vi "Autonomous Independent (1).vi"() -> ()   [LabVIEW 2017]
doc: "This VI is called when autonomous begins, and will automatically be terminated when autonomous ends. You can carry out timed or sensor driven robot movement independently without needing to return to the caller."
uses:
  <vilib>/Rock Robotics/WPI/ThirdParty/Sensors/navX/_TypeDefs/FRIC_navX_DeviceNumbersTypeDef.ctl
  Public/Documents/Cross The Road Electronics/Phoenix-LabVIEW/Motor Controller/Controls/CTRE_Phoenix_MotorControl_ControlMode.ctl
  <vilib>/Rock Robotics/WPI/Utilities/WPI_GetSetVariantRefNum.vi
  <vilib>/Rock Robotics/Network Tables/NT Read String.vi
  <vilib>/Rock Robotics/Network Tables/NT Write Numeric Array.vi
panel:
  out "error out":errorcluster
  out "Array":dbl[](array[numeric])
  out "Direction":string[](array[string])
  in  "Target Angle":dbl format="%#_13g"
  in  "Target Distance":dbl=500.0 format="%#_13g"
  # "Be sure to right-click and choose Data Operations>>Make Current Value default if you want to save the array values with the VI"
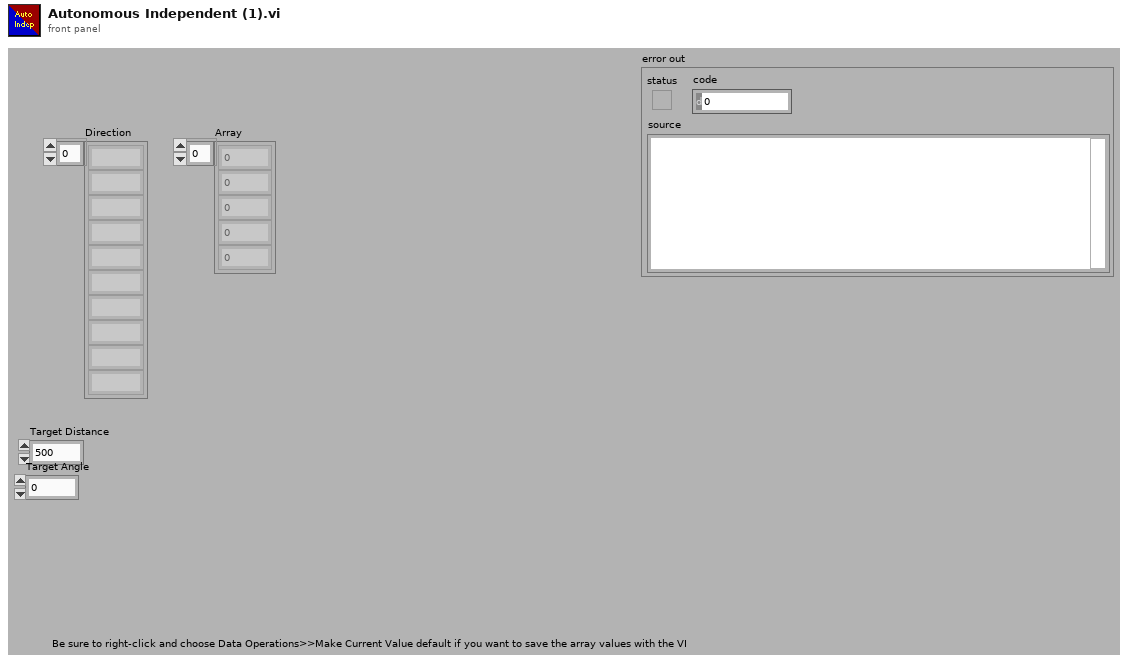
[diagram p1: front panel]
types:
  T1 = typedef "FRIC_navX_DeviceNumbersTypeDef.ctl" = enum16{"Dev0", "Dev1", "Dev2", "Dev3"}
  T2 = cluster{"Left Encoder":string, "Right Encoder":string, "Gyro Refnum":string, "Device Number":T1, "Right Refnum":string, "Left Refnum":string, "Right Intake":string, "Left Intake":string}
  T3 = typedef "WPI_JoystickDevRef.ctl" = cluster{"Device":T4}
  T4 = typedef "WPI_JoystickDeviceEnum.ctl" = enum16{"USB 0", "USB 1", "USB 2", "USB 3", "USB 4", "USB 5"}
  T5 = cluster{"Left Encoder":string, "Right Encoder":string, "Gyro Refnum":string, "Device Number":T1, "Right Refnum":string, "Left Refnum":string}
  T6 = cluster{"Left Encoder":string, "Right Encoder":string, "Gyro Refnum":string, "Device Number":T1, "Right Refnum":string, "Left Refnum":string, "Left Intake":string, "Right Intake":string}
  T7 = typedef "CTRE_Phoenix_MotorControl_ControlMode.ctl" = u16
  T8 = typedef "WPI_MotorControlDeviceRef.ctl" = cluster{"DeviceStatus":errorcluster, "Type":T9, "PWM":cluster{"PWM Channel":T10, "DeadBand":T11}, "CAN":cluster{"Device Number":u8, "SetOutput VI Ref":variant, "GetOutput VI Ref":variant, "Enable VI Ref":variant, "Disable VI Ref":variant, "Data":variant}, "Invert":bool, "DIO PWM":cluster{"PWM \"Enable\" Channel":T10, "DIOChannel":T12, "PWM Rate":dbl}}
  T9 = typedef "WPI_MotorControlType.ctl" = enum16{"PWM", "CAN", "DIO PWM"}
  T10 = typedef "FPGA_DIOPWMChannel.ctl" = enum8{"PWM 0", "PWM 1", "PWM 2", "PWM 3", "PWM 4", "PWM 5", "PWM 6", "PWM 7", "PWM 8", "PWM 9", "PWM MXP 0", "PWM MXP 1", "PWM MXP 2", "PWM MXP 3", "PWM MXP 4", "PWM MXP 5", "PWM MXP 6", "PWM MXP 7", "PWM MXP 8", "PWM MXP 9", "Invalid"}
  T11 = typedef "WPI_PWMDeadband.ctl" = cluster{"Name":string, "maxPositivePwm":i32, "minPositivePwm":i32, "centerPwm":i32, "maxNegativePwm":i32, "minNegativePwm":i32, "angularRange":u16}
  T12 = typedef "FPGA_DIOChannel.ctl" = enum8{"DIO 0", "DIO 1", "DIO 2", "DIO 3", "DIO 4", "DIO 5", "DIO 6", "DIO 7", "DIO 8", "DIO 9", "DIO MXP 0", "DIO MXP 1", "DIO MXP 2", "DIO MXP 3", "DIO MXP 4", "DIO MXP 5", "DIO MXP 6", "DIO MXP 7", "DIO MXP 8", "DIO MXP 9", "DIO MXP 10", "DIO MXP 11", "DIO MXP 12", "DIO MXP 13", "DIO MXP 14", "DIO MXP 15", "SPI Port CS1", "SPI Port CS2", "SPI Port CS3", "SPI Port MISO", "SPI Port MOSI", "Invalid"}
  T13 = cluster{"Width":u16, "Style":enum32{"Solid", "Dash", "Dot", "DashDot", "DashDotDot"}}
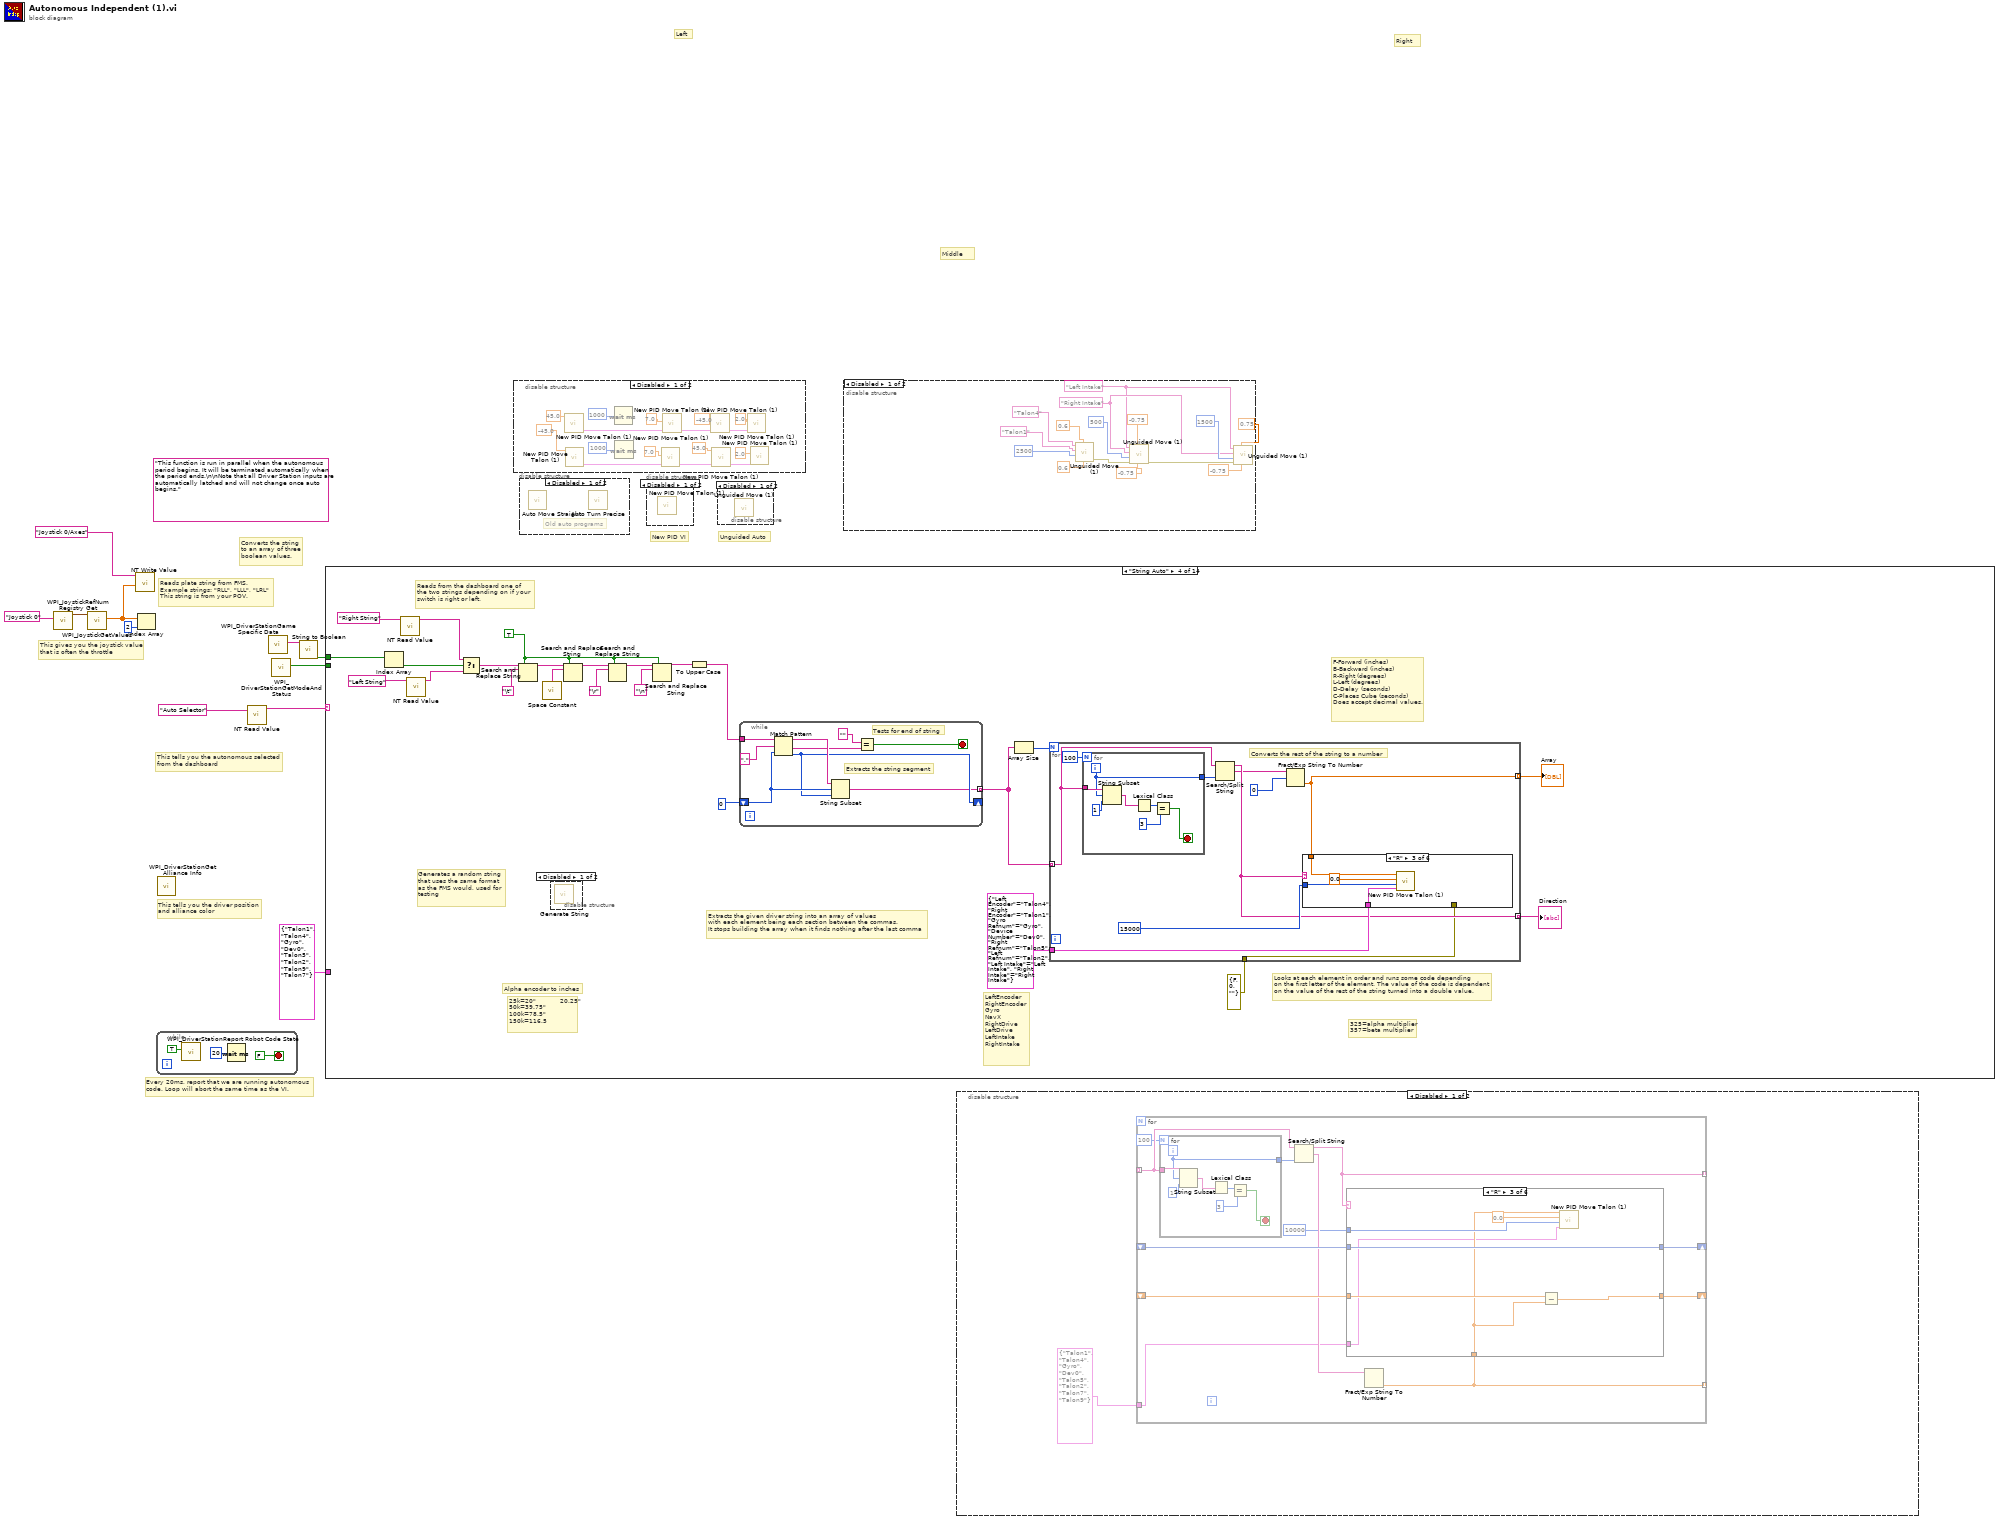
[diagram p0: block diagram]
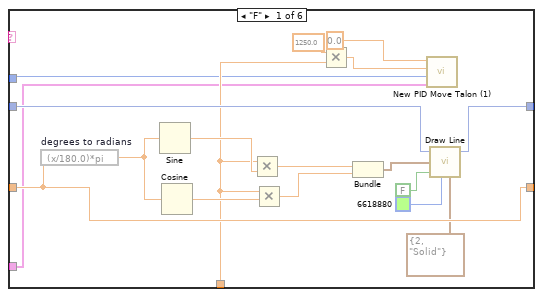
[diagram p2: hidden frame]
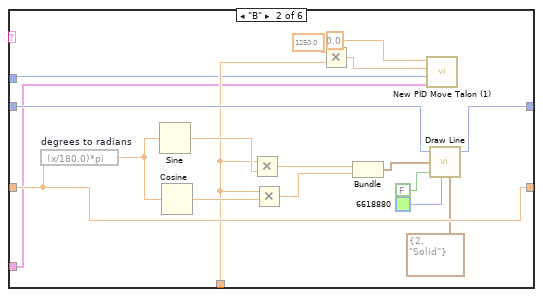
[diagram p3: hidden frame]
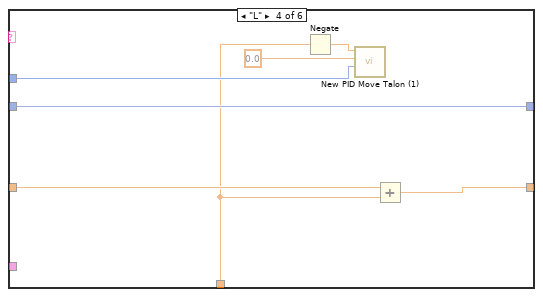
[diagram p4: hidden frame]
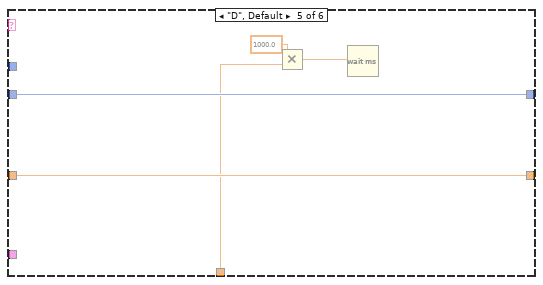
[diagram p5: hidden frame]
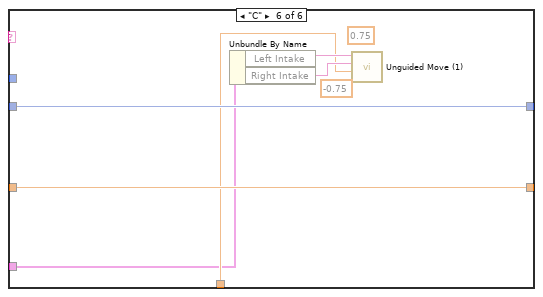
[diagram p6: hidden frame]
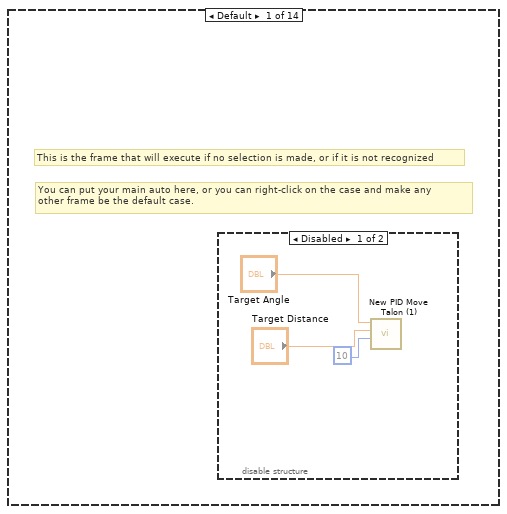
[diagram p13: hidden frame]
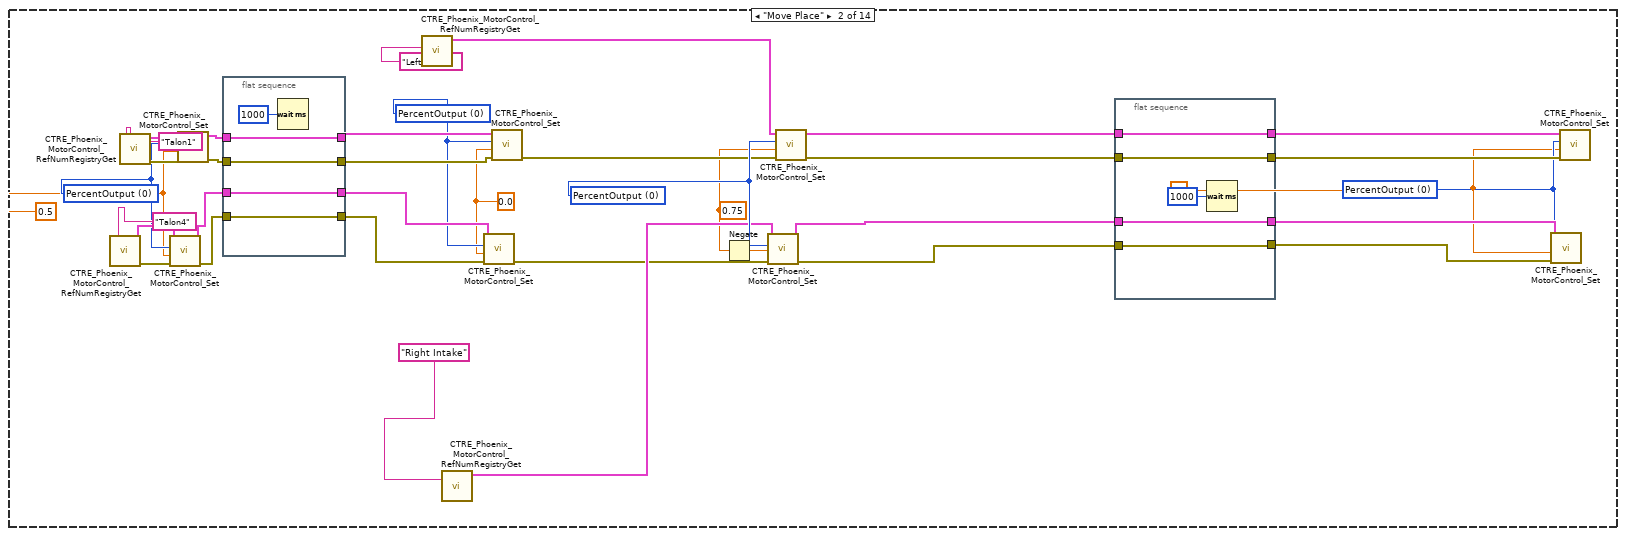
[diagram p15: hidden frame]
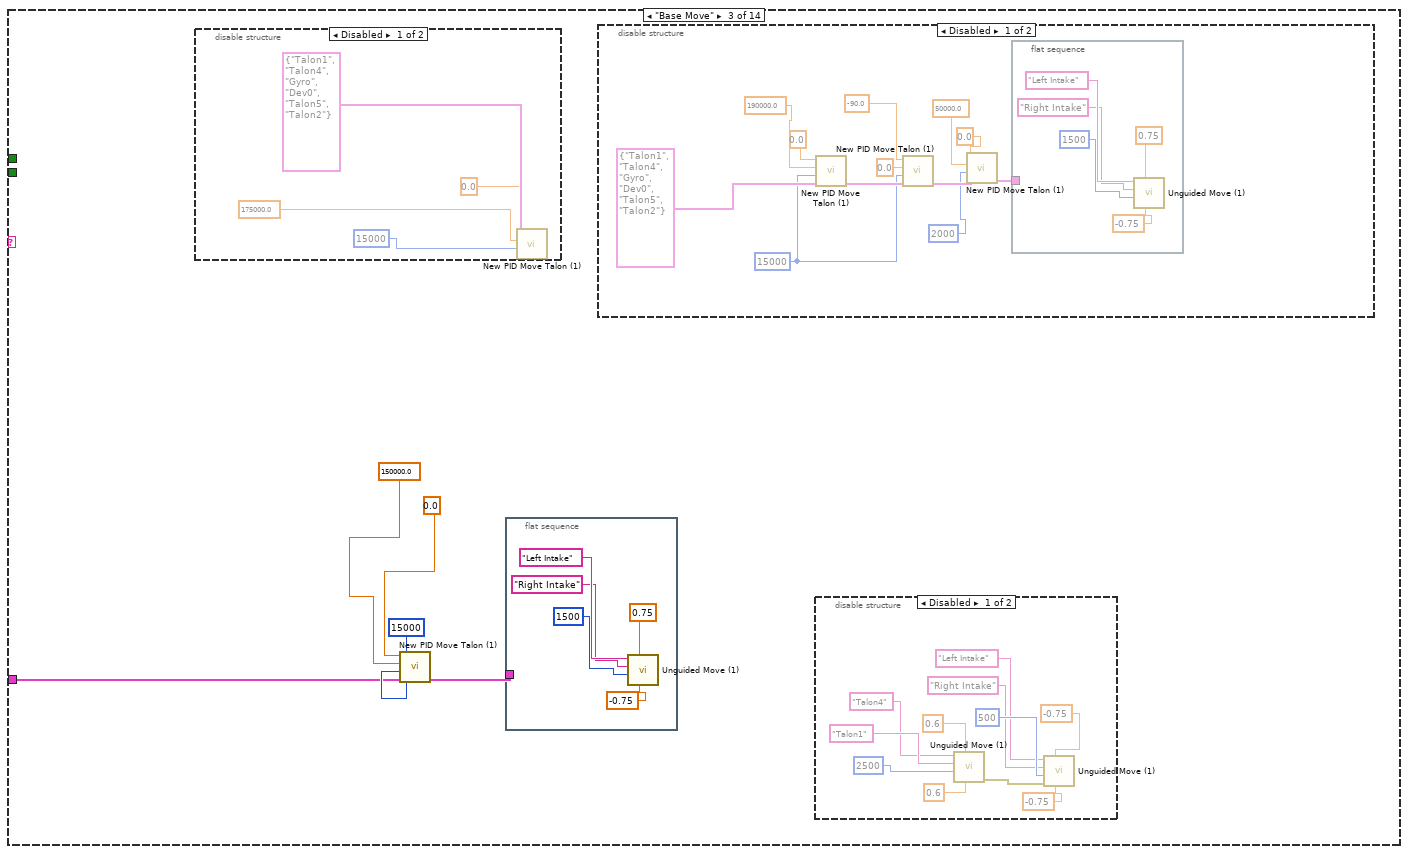
[diagram p16: hidden frame]
diagram:
  (unwired) "This function is run in parallel when the autonomous period begins. It will be terminated automatically when the period ends.\n\nNote that all Driver Station inputs are automatically latched and will not change once auto begins."
  # "Unguided Auto"
  # "New PID VI"
  # "Converts the string\nto an array of three\nboolean values."
  # "Reads plate string from FMS. \nExample strings: \"RLL\", \"LLL\", \"LRL\"\nThis string is from your POV."
  # "Middle"
  # "Left"
  # "Right"
  # "This tells you the autonomous selected\nfrom the dashboard"
  # "Every 20ms, report that we are running autonomous\ncode. Loop will abort the same time as the VI."
  # "This gives you the joystick value\nthat is often the throttle"
  # "This tells you the driver position\nand alliance color"
  n1 = call <vilib>:"WPI_JoystickRefNum Registry Get.vi"("refnum name"="Joystick 0") -> ("JoystickDevRef"=w10:T3)  [unwired: 1 in, 9 out]
  n2 = call <vilib>:"WPI_JoystickGetValues.vi"("JoystickDevRef"=w10) -> ("Axes"=w6:dbl[])  [unwired: 6 in, 4 out]
  n3 = call-poly <vilib>:"NT Write Value.vi"("Numeric Array"=w6, "Name"="Joystick 0/Axes") -> ()  [unwired: 9 in, 1 out]
  n4 = Index Array(array=w6, index=2) -> ()  [unwired: 1 out]
  n5 = while {
    stop <- FALSE stop-if-true
    n6 = call <vilib>:"WPI_DriverStationReport Robot Code State.vi"("Autonomous"=TRUE) -> ()  [unwired: 10 in, 1 out]
    n7 = Wait (ms)(milliseconds to wait=u32 20) -> ()  [unwired: 1 out]
  }
  n8 = call <vilib>:"WPI_DriverStationGet Alliance Info.vi"() -> ()  [unwired: 12 out]
  n9 = call-poly <vilib>:"NT Read Value.vi"("Name"="Auto Selector") -> ("String"=w7:string)  [unwired: 9 in, 1 out]
  n10 = call <vilib>:"WPI_DriverStationGame Specific Data.vi"() -> ("Game Specific Data"=w3:string)  [unwired: 11 in]
  n11 = call <vilib>:"WPI_DriverStationGetModeAndStatus.vi"() -> ("FMS Attached"=w4:bool)  [unwired: 10 in, 1 out]
  n12 = call "String to Boolean.vi"("String"=w3) -> ("Boolean Array"=w2:bool[])  [unwired: 10 in]
  n13 = case shown="\"String Auto\"" w7 {
    tunnel: w4 -> [_ _ _ _ _ _ _ _ _ _ _ _ _ _]
    tunnel: w2 -> [_ _ _ w119 w194 _ _ w242 _ _ _ _ _ _]
    tunnel: T2 {"Left Encoder"="Talon1", "Right Encoder"="Talon4", "Gyro Refnum"="Gyro", "Device Number"=enum."Dev0", "Right Refnum"="Talon5", "Left Refnum"="Talon2", "Right Intake"="Talon9", "Left Intake"="Talon7"} ("Cluster 3") -> [_ _ w65 _ _ _ _ _ _ _ _ _ _ _]
    frame Default {
      # "You can put your main auto here, or you can right-click on the case and make any\nother frame be the default case."
      # "This is the frame that will execute if no selection is made, or if it is not recognized"
      n14 = disable-structure shown="Disabled" {
        frame Disabled {
          n15 = call "New PID Move Talon (1).vi"("Timeout"=i8 10, "Target Distance"="Target Distance", "Target Angle"="Target Angle") -> ()  [unwired: 8 in, 1 out]
        }
        frame Enabled {
        }
      }
    }
    frame "Move Place" {
      w20 = 0.0 ("Output")
      w21 = T7 0 items=["PercentOutput"=0, "Position"=1, "Velocity"=2, "Current"=3, "Follower"=5, "MotionProfile"=6, "MotionMagic"=7, "MotionMagicArc"=8, "MotionProfileArc"=10, "Disabled"=15] ("Control Mode")
      w19 = 0.75 ("Output")
      w36 = T7 0 items=["PercentOutput"=0, "Position"=1, "Velocity"=2, "Current"=3, "Follower"=5, "MotionProfile"=6, "MotionMagic"=7, "MotionMagicArc"=8, "MotionProfileArc"=10, "Disabled"=15] ("Control Mode")
      w37 = 0.0 ("Output")
      w38 = T7 0 items=["PercentOutput"=0, "Position"=1, "Velocity"=2, "Current"=3, "Follower"=5, "MotionProfile"=6, "MotionMagic"=7, "MotionMagicArc"=8, "MotionProfileArc"=10, "Disabled"=15] ("Control Mode")
      w47 = 0.5 ("Output")
      w48 = T7 0 items=["PercentOutput"=0, "Position"=1, "Velocity"=2, "Current"=3, "Follower"=5, "MotionProfile"=6, "MotionMagic"=7, "MotionMagicArc"=8, "MotionProfileArc"=10, "Disabled"=15] ("Control Mode")
      n16 = call <vilib>:"CTRE_Phoenix_MotorControl_RefNumRegistryGet.vi"("refnum name"="Talon4") -> ("error out"=w49:errorcluster, "PhoenixMotorControlDevRef"=w50:T8)  [unwired: 9 in]
      n17 = call <vilib>:"CTRE_Phoenix_MotorControl_RefNumRegistryGet.vi"("refnum name"="Talon1") -> ("error out"=w52:errorcluster, "PhoenixMotorControlDevRef"=w51:T8)  [unwired: 9 in]
      n18 = call <vilib>:"CTRE_Phoenix_MotorControl_Set.vi"("error in (no error)"=w49, "Output"=w47, "Control Mode"=w48, "PhoenixMotorControlDevRef"=w50) -> ("error out"=w43:errorcluster, "PhoenixMotorControlDevRef"=w44:T8)  [unwired: 6 in]
      n19 = call <vilib>:"CTRE_Phoenix_MotorControl_Set.vi"("error in (no error)"=w52, "Output"=w47, "Control Mode"=w48, "PhoenixMotorControlDevRef"=w51) -> ("error out"=w45:errorcluster, "PhoenixMotorControlDevRef"=w46:T8)  [unwired: 6 in]
      n20 = flat-sequence {
        tunnel: w46 -> [w64]
        tunnel: [w64] -> w42
        tunnel: [w63] -> w40
        tunnel: w44 -> [w63]
        tunnel: [w62] -> w39
        tunnel: w43 -> [w62]
        tunnel: w45 -> [w61]
        tunnel: [w61] -> w41
        frame #0 {
          n21 = Wait (ms)(milliseconds to wait=u32 1000) -> ()  [unwired: 1 out]
        }
      }
      n22 = call <vilib>:"CTRE_Phoenix_MotorControl_RefNumRegistryGet.vi"("refnum name"="Left Intake") -> ("PhoenixMotorControlDevRef"=w35:T8)  [unwired: 9 in, 1 out]
      n23 = call <vilib>:"CTRE_Phoenix_MotorControl_RefNumRegistryGet.vi"("refnum name"="Right Intake") -> ("PhoenixMotorControlDevRef"=w34:T8)  [unwired: 9 in, 1 out]
      n24 = call <vilib>:"CTRE_Phoenix_MotorControl_Set.vi"("error in (no error)"=w39, "Output"=w37, "Control Mode"=w38, "PhoenixMotorControlDevRef"=w40) -> ("error out"=w33:errorcluster)  [unwired: 6 in, 1 out]
      n25 = call <vilib>:"CTRE_Phoenix_MotorControl_Set.vi"("error in (no error)"=w41, "Output"=w37, "Control Mode"=w38, "PhoenixMotorControlDevRef"=w42) -> ("error out"=w32:errorcluster)  [unwired: 6 in, 1 out]
      n26 = Negate(x=w19) -> (-x=w18:dbl)
      n27 = call <vilib>:"CTRE_Phoenix_MotorControl_Set.vi"("error in (no error)"=w33, "Output"=w18, "Control Mode"=w36, "PhoenixMotorControlDevRef"=w34) -> ("error out"=w29:errorcluster, "PhoenixMotorControlDevRef"=w26:T8)  [unwired: 6 in]
      n28 = call <vilib>:"CTRE_Phoenix_MotorControl_Set.vi"("error in (no error)"=w32, "Output"=w19, "Control Mode"=w36, "PhoenixMotorControlDevRef"=w35) -> ("error out"=w28:errorcluster, "PhoenixMotorControlDevRef"=w27:T8)  [unwired: 6 in]
      n29 = flat-sequence {
        tunnel: [w59] -> w22
        tunnel: w29 -> [w59]
        tunnel: [w58] -> w24
        tunnel: w28 -> [w58]
        tunnel: [w57] -> w25
        tunnel: w27 -> [w57]
        tunnel: [w56] -> w23
        tunnel: w26 -> [w56]
        frame #0 {
          n30 = Wait (ms)(milliseconds to wait=u32 1000) -> ()  [unwired: 1 out]
        }
      }
      n31 = call <vilib>:"CTRE_Phoenix_MotorControl_Set.vi"("error in (no error)"=w22, "Output"=w20, "Control Mode"=w21, "PhoenixMotorControlDevRef"=w23) -> ()  [unwired: 6 in, 2 out]
      n32 = call <vilib>:"CTRE_Phoenix_MotorControl_Set.vi"("error in (no error)"=w24, "Output"=w20, "Control Mode"=w21, "PhoenixMotorControlDevRef"=w25) -> ()  [unwired: 6 in, 2 out]
    }
    frame "Base Move" {
      n33 = disable-structure shown="Disabled" {
        frame Disabled {
          n34 = call "New PID Move Talon (1).vi"("Cluster 3"=T5 {"Left Encoder"="Talon1", "Right Encoder"="Talon4", "Gyro Refnum"="Gyro", "Device Number"=enum."Dev0", "Right Refnum"="Talon5", "Left Refnum"="Talon2"}, "Timeout"=i16 15000, "Target Distance"=175000.0 ("Target Distance 2"), "Target Angle"=0.0) -> ()  [unwired: 7 in, 1 out]
        }
        frame Enabled {
        }
      }
      n35 = call "New PID Move Talon (1).vi"("Cluster 3"=w65, "Timeout"=i16 15000, "Target Distance"=150000.0, "Target Angle"=0.0) -> ("Cluster 2"=w66:T2)  [unwired: 7 in]
      n36 = flat-sequence {
        tunnel: w66 -> [_]
        frame #0 {
          n37 = call "Unguided Move (1).vi"("Power 2"=-0.75 ("Power"), "Power"=0.75, "milliseconds to wait"=u32 1500, "refnum name 2"="Right Intake" ("refnum name"), "refnum name"="Left Intake") -> ()  [unwired: 6 in, 1 out]
        }
      }
      n38 = disable-structure shown="Disabled" {
        frame Disabled {
          w82 = i16 15000 ("Timeout")
          n39 = call "New PID Move Talon (1).vi"("Cluster 3"=T5 {"Left Encoder"="Talon1", "Right Encoder"="Talon4", "Gyro Refnum"="Gyro", "Device Number"=enum."Dev0", "Right Refnum"="Talon5", "Left Refnum"="Talon2"}, "Timeout"=w82, "Target Distance"=190000.0, "Target Angle"=0.0) -> ("Cluster 2"=w86:T2)  [unwired: 7 in]
          n40 = call "New PID Move Talon (1).vi"("Cluster 3"=w86, "Timeout"=w82, "Target Distance"=0.0, "Target Angle"=-90.0) -> ("Cluster 2"=w85:T2)  [unwired: 7 in]
          n41 = call "New PID Move Talon (1).vi"("Cluster 3"=w85, "Timeout"=i16 2000, "Target Distance"=50000.0, "Target Angle"=0.0) -> ("Cluster 2"=w84:T2)  [unwired: 7 in]
          n42 = flat-sequence {
            tunnel: w84 -> [_]
            frame #0 {
              n43 = call "Unguided Move (1).vi"("Power 2"=-0.75 ("Power"), "Power"=0.75, "milliseconds to wait"=u32 1500, "refnum name 2"="Right Intake" ("refnum name"), "refnum name"="Left Intake") -> ()  [unwired: 6 in, 1 out]
            }
          }
        }
        frame Enabled {
        }
      }
      n44 = disable-structure shown="Disabled" {
        frame Disabled {
          n45 = call "Unguided Move (1).vi"("Power 2"=0.6, "Power"=0.6, "milliseconds to wait"=u32 2500, "refnum name 2"="Talon1", "refnum name"="Talon4") -> ("error out"=w102:errorcluster)  [unwired: 6 in]
          n46 = call "Unguided Move (1).vi"("Power 2"=-0.75 ("Power"), "Power"=-0.75, "error in (no error)"=w102, "milliseconds to wait"=u32 500, "refnum name 2"="Right Intake" ("refnum name"), "refnum name"="Left Intake") -> ()  [unwired: 5 in, 1 out]
        }
        frame Enabled {
        }
      }
    }
    frame "String Auto" {
      w111 = TRUE ("replace all? (F)")
      # "325=alpha multiplier\n357=beta multiplier"
      # "F-Forward (inches)\nB-Backward (inches)\nR-Right (degrees)\nL-Left (degrees)\nD-Delay (seconds)\nC-Places Cube (seconds)\nDoes accept decimal values."
      # "Alpha encoder to inches"
      # "LeftEncoder\nRightEncoder\nGyro\nNavX\nRightDrive\nLeftDrive\nLeftIntake\nRightIntake"
      # "25k=20\"            20.25\"\n50k=39.75\"\n100k=78.5\"\n150k=116.5"
      # "Looks at each element in order and runs some code depending\non the first letter of the element. The value of the code is dependent\non the value of the rest of the string turned into a double value."
      # "Extracts the given driver string into an array of values \nwith each element being each section between the commas.\nIt stops building the array when it finds nothing after the last comma"
      # "Reads from the dashboard one of\nthe two strings depending on if your\nswitch is right or left."
      # "Generates a random string\nthat uses the same format \nas the FMS would, used for\ntesting"
      n47 = Index Array(array=w119) -> (element=w130:bool)  [unwired: 1 in]
      n48 = call-poly <vilib>:"NT Read Value.vi"("Name"="Right String") -> ("String"=w129:string)  [unwired: 9 in, 1 out]
      n49 = call-poly <vilib>:"NT Read Value.vi"("Name"="Left String") -> ("String"=w126:string)  [unwired: 9 in, 1 out]
      n50 = Select(t=w129, s=w130, f=w126) -> (s? t:f=w109:string)
      n51 = Search and Replace String(replace all?=w111, input string=w109, search string="\t") -> (result string=w115:string)  [unwired: 5 in, 3 out]
      n52 = call <vilib>:"Space Constant.vi"() -> ("String"=w113:string)
      n53 = disable-structure shown="Disabled" {
        frame Disabled {
          n54 = call "Generate String.vi"() -> ()  [unwired: 11 in, 1 out]
        }
        frame Enabled {
        }
      }
      n55 = Search and Replace String(replace all?=w111, input string=w115, search string=w113) -> (result string=w116:string)  [unwired: 5 in, 3 out]
      n56 = Search and Replace String(replace all?=w111, input string=w116, search string="\r") -> (result string=w117:string)  [unwired: 5 in, 3 out]
      n57 = Search and Replace String(replace all?=w111, input string=w117, search string="\n") -> (result string=w110:string)  [unwired: 5 in, 3 out]
      n58 = To Upper Case(1:w110) -> (0:w108:string)
      n59 = while {
        tunnel: w108 -> [w191]
        shift-right: [w187] -> _
        shift-left: 0 ("offset past match") -> [w188]
        tunnel: [w186] -> w123 mode=indexing
        stop <- w183 stop-if-true
        # "Tests for end of string"
        # "Extracts the string segment"
        n60 = Match Pattern(string=w191, regular expression=",", offset (0)=w188) -> (before substring=w189:string, after substring=w185:string, offset past match=w187:i32)  [unwired: 1 out]
        n61 = String Subset(string=w189, offset (0)=w188, length (rest)=w187) -> (substring=w186:string)
        n62 = Equal?(x="", y=w185) -> (x = y?=w183:bool)
      }
      n63 = Array Size(array=w123) -> (size(s)=w124:i32)
      n64 = for {
        N: w124 -> [_]
        tunnel: w123 -> [w135] mode=indexing
        tunnel: [w139] -> w121 mode=indexing
        tunnel: [w134] -> w122 mode=indexing
        tunnel: T6 {"Left Encoder"="Talon4", "Right Encoder"="Talon1", "Gyro Refnum"="Gyro", "Device Number"=enum."Dev0", "Right Refnum"="Talon5", "Left Refnum"="Talon2", "Left Intake"="Left Intake", "Right Intake"="Right Intake"} ("Cluster 3") -> [w138]
        tunnel: errorcluster {"status"=FALSE, "code"=0, "source"=""} ("error in (no error)") -> [w131]
        # "Converts the rest of the string to a number"
        n65 = for {
          N: 100 -> [_]
          tunnel: w135 -> [w145]
          tunnel: [w142] -> w136
          i -> [w142]
          stop <- w141 stop-if-true
          n66 = String Subset(string=w145, offset (0)=w142, length (rest)=1 ("length (rest)")) -> (substring=w143:string)
          n67 = Lexical Class(1:w143) -> (0:w147:i16)
          n68 = Equal?(x=w147, y=i16 3) -> (x = y?=w141:bool)
        }
        n69 = Search/Split String(string=w135, offset (0)=w136) -> (substring before match=w134:string, match + rest of string=w133:string)  [unwired: 1 in, 1 out]
        n70 = Fract/Exp String To Number(string=w133, offset=0) -> (number=w139:dbl)  [unwired: 2 in, 1 out]
        n71 = case shown="\"R\"" w134 {
          tunnel: w139 -> [w149 w157 w164 w167 w171 w181]
          tunnel: w138 -> [w153 w160 w162 w166 _ w182]
          tunnel: i16 15000 ("Timeout") -> [w152 w159 w161 w165 _ _]
          tunnel: w131 -> [_ _ _ _ _ w173]
          frame "F", Default {
            n72 = Multiply(x=325.0, y=w149) -> (x*y=w148:dbl)
            n73 = call "New PID Move Talon (1).vi"("Cluster 3"=w153, "Timeout"=w152, "Target Distance"=w148, "Target Angle"=0.0) -> ()  [unwired: 7 in, 1 out]
          }
          frame "B" {
            n74 = Negate(x=w157) -> (-x=w156:dbl)
            n75 = Multiply(x=1250.0, y=w156) -> (x*y=w155:dbl)
            n76 = call "New PID Move Talon (1).vi"("Cluster 3"=w160, "Timeout"=w159, "Target Distance"=w155, "Target Angle"=0.0) -> ()  [unwired: 7 in, 1 out]
          }
          frame "R" {
            n77 = call "New PID Move Talon (1).vi"("Cluster 3"=w162, "Timeout"=w161, "Target Distance"=0.0, "Target Angle"=w164) -> ()  [unwired: 7 in, 1 out]
          }
          frame "L" {
            n78 = Negate(x=w167) -> (-x=w168:dbl)
            n79 = call "New PID Move Talon (1).vi"("Cluster 3"=w166, "Timeout"=w165, "Target Distance"=0.0, "Target Angle"=w168) -> ()  [unwired: 7 in, 1 out]
          }
          frame "D" {
            n80 = Multiply(x=1000.0, y=w171) -> (x*y=w170:dbl)
            n81 = Wait (ms)(milliseconds to wait=w170) -> ()  [unwired: 1 out]
          }
          frame "C" {
            n82 = Multiply(x=w181, y=1000.0) -> (x*y=w177:dbl)
            n83 = Unbundle By Name(w182) -> ("Left Intake"=w178:string, "Right Intake"=w179:string)
            n84 = call "Unguided Move (1).vi"("Power 2"=-0.75, "Power"=0.75, "error in (no error)"=w173, "milliseconds to wait"=w177, "refnum name 2"=w179, "refnum name"=w178) -> ("error out"=→"error out":errorcluster)  [unwired: 5 in]
          }
        }
      }
      "Direction" <- w122
      "Array" <- w121
    }
    frame "Front Left Auto" {
      w197 = "Right Intake" ("refnum name")
      w195 = "Left Intake" ("refnum name")
      n85 = Index Array(array=w194) -> (element=w193:bool)  [unwired: 1 in]
      n86 = Not(x=w193) -> (.not. x?=w192:bool)
      n87 = call "Unguided Move (1).vi"("Power 2"=0.6, "Power"=0.6, "milliseconds to wait"=u32 2500, "refnum name 2"="Talon1", "refnum name"="Talon4") -> ("error out"=w199:errorcluster)  [unwired: 6 in]
      n88 = call "Unguided Move (1).vi"("Power 2"=-0.75 ("Power"), "Power"=-0.75, "error in (no error)"=w199, "milliseconds to wait"=u32 500, "refnum name 2"=w197, "refnum name"=w195) -> ("error out"=w196:errorcluster)  [unwired: 5 in]
      n89 = case shown="True" w192 {
        tunnel: w197 -> [_ w212]
        tunnel: w196 -> [_ w209]
        tunnel: w195 -> [_ w208]
        frame False {
        }
        frame True {
          n90 = call "Unguided Move (1).vi"("Power 2"=-0.75, "Power"=0.75, "error in (no error)"=w209, "milliseconds to wait"=u32 1500, "refnum name 2"=w212, "refnum name"=w208) -> ()  [unwired: 5 in, 1 out]
        }
      }
      n91 = disable-structure shown="Enabled" {
        frame Disabled {
          n92 = call "New PID Move Talon (1).vi"("Target Distance"=4.0 ("Target Angle")) -> ("Cluster 2"=w219:T2)  [unwired: 10 in]
          n93 = call "New PID Move Talon (1).vi"("Cluster 3"=w219, "Target Angle"=90.0 ("Target Distance")) -> ("Cluster 2"=w220:T2)  [unwired: 9 in]
          n94 = call "New PID Move Talon (1).vi"("Cluster 3"=w220, "Target Distance"=5.0 ("Target Angle")) -> ("Cluster 2"=w218:T2)  [unwired: 9 in]
          n95 = call "New PID Move Talon (1).vi"("Cluster 3"=w218, "Target Angle"=-90.0 ("Target Distance")) -> ("Cluster 2"=w221:T2)  [unwired: 9 in]
          n96 = call "New PID Move Talon (1).vi"("Cluster 3"=w221, "Target Distance"=5.0) -> ()  [unwired: 9 in, 1 out]
        }
        frame Enabled {
        }
      }
    }
    frame "Side Left Auto" {
      w222 = i16 15000 ("Timeout")
      n97 = call "New PID Move Talon (1).vi"("Timeout"=w222, "Target Distance"=150000.0) -> ("Cluster 2"=w227:T2)  [unwired: 9 in]
      n98 = call "New PID Move Talon (1).vi"("Cluster 3"=w227, "Timeout"=w222, "Target Angle"=90.0) -> ("Cluster 2"=w226:T2)  [unwired: 8 in]
      n99 = call "New PID Move Talon (1).vi"("Cluster 3"=w226, "Timeout"=w222, "Target Distance"=10000.0) -> ()  [unwired: 8 in, 1 out]
    }
    frame "Other Side Left Auto" {
      n100 = call "New PID Move Talon (1).vi"("Target Distance"=18.5 ("Target Angle")) -> ("Cluster 2"=w236:T2)  [unwired: 10 in]
      n101 = call "New PID Move Talon (1).vi"("Cluster 3"=w236, "Target Angle"=90.0 ("Target Distance")) -> ("Cluster 2"=w237:T2)  [unwired: 9 in]
      n102 = call "New PID Move Talon (1).vi"("Cluster 3"=w237, "Target Distance"=18.0 ("Target Angle")) -> ("Cluster 2"=w235:T2)  [unwired: 9 in]
      n103 = call "New PID Move Talon (1).vi"("Cluster 3"=w235, "Target Angle"=90.0 ("Target Distance")) -> ("Cluster 2"=w238:T2)  [unwired: 9 in]
      n104 = call "New PID Move Talon (1).vi"("Cluster 3"=w238, "Target Distance"=5.0) -> ("Cluster 2"=w239:T2)  [unwired: 9 in]
      n105 = call "New PID Move Talon (1).vi"("Cluster 3"=w239, "Target Angle"=90.0) -> ("Cluster 2"=w240:T2)  [unwired: 9 in]
      n106 = call "New PID Move Talon (1).vi"("Cluster 3"=w240, "Target Distance"=1.0) -> ()  [unwired: 9 in, 1 out]
    }
    frame "Front Right Auto" {
      w245 = "Right Intake" ("refnum name")
      w243 = "Left Intake" ("refnum name")
      n107 = Index Array(array=w242) -> (element=w241:bool)  [unwired: 1 in]
      n108 = call "Unguided Move (1).vi"("Power 2"=0.6, "Power"=0.6, "milliseconds to wait"=u32 2500, "refnum name 2"="Talon2", "refnum name"="Talon5") -> ("error out"=w247:errorcluster)  [unwired: 6 in]
      n109 = call "Unguided Move (1).vi"("Power 2"=-0.75 ("Power"), "Power"=-0.75, "error in (no error)"=w247, "milliseconds to wait"=u32 500, "refnum name 2"=w245, "refnum name"=w243) -> ("error out"=w244:errorcluster)  [unwired: 5 in]
      n110 = case shown="True" w241 {
        tunnel: w245 -> [_ w260]
        tunnel: w244 -> [_ w257]
        tunnel: w243 -> [_ w256]
        frame False {
        }
        frame True {
          n111 = call "Unguided Move (1).vi"("Power 2"=-0.75, "Power"=0.75, "error in (no error)"=w257, "milliseconds to wait"=u32 1500, "refnum name 2"=w260, "refnum name"=w256) -> ()  [unwired: 5 in, 1 out]
        }
      }
      n112 = disable-structure shown="Disabled" {
        frame Disabled {
          n113 = call "New PID Move Talon (1).vi"("Target Distance"=4.0 ("Target Angle")) -> ("Cluster 2"=w267:T2)  [unwired: 10 in]
          n114 = call "New PID Move Talon (1).vi"("Cluster 3"=w267, "Target Angle"=-90.0 ("Target Distance")) -> ("Cluster 2"=w268:T2)  [unwired: 9 in]
          n115 = call "New PID Move Talon (1).vi"("Cluster 3"=w268, "Target Distance"=5.0 ("Target Angle")) -> ("Cluster 2"=w266:T2)  [unwired: 9 in]
          n116 = call "New PID Move Talon (1).vi"("Cluster 3"=w266, "Target Angle"=90.0 ("Target Distance")) -> ("Cluster 2"=w269:T2)  [unwired: 9 in]
          n117 = call "New PID Move Talon (1).vi"("Cluster 3"=w269, "Target Distance"=5.0) -> ()  [unwired: 9 in, 1 out]
        }
        frame Enabled {
        }
      }
    }
    frame "Side Right Auto" {
      n118 = call "New PID Move Talon (1).vi"("Target Distance"=12.0) -> ("Cluster 2"=w274:T2)  [unwired: 10 in]
      n119 = call "New PID Move Talon (1).vi"("Cluster 3"=w274, "Target Angle"=-90.0) -> ("Cluster 2"=w273:T2)  [unwired: 9 in]
      n120 = call "New PID Move Talon (1).vi"("Cluster 3"=w273, "Target Distance"=1.5) -> ()  [unwired: 9 in, 1 out]
    }
    frame "Other Side Right Auto" {
      n121 = call "New PID Move Talon (1).vi"("Target Distance"=18.5 ("Target Angle")) -> ("Cluster 2"=w283:T2)  [unwired: 10 in]
      n122 = call "New PID Move Talon (1).vi"("Cluster 3"=w283, "Target Angle"=-90.0 ("Target Distance")) -> ("Cluster 2"=w284:T2)  [unwired: 9 in]
      n123 = call "New PID Move Talon (1).vi"("Cluster 3"=w284, "Target Distance"=18.0 ("Target Angle")) -> ("Cluster 2"=w282:T2)  [unwired: 9 in]
      n124 = call "New PID Move Talon (1).vi"("Cluster 3"=w282, "Target Angle"=-90.0 ("Target Distance")) -> ("Cluster 2"=w285:T2)  [unwired: 9 in]
      n125 = call "New PID Move Talon (1).vi"("Cluster 3"=w285, "Target Distance"=5.0) -> ("Cluster 2"=w286:T2)  [unwired: 9 in]
      n126 = call "New PID Move Talon (1).vi"("Cluster 3"=w286, "Target Angle"=-90.0) -> ("Cluster 2"=w287:T2)  [unwired: 9 in]
      n127 = call "New PID Move Talon (1).vi"("Cluster 3"=w287, "Target Distance"=1.0) -> ()  [unwired: 9 in, 1 out]
    }
    frame "Middle Left Side Auto" {
      n128 = call "New PID Move Talon (1).vi"("Target Distance"=5.0) -> ("Cluster 2"=w294:T2)  [unwired: 10 in]
      n129 = call "New PID Move Talon (1).vi"("Cluster 3"=w294, "Target Angle"=-90.0) -> ("Cluster 2"=w295:T2)  [unwired: 9 in]
      n130 = call "New PID Move Talon (1).vi"("Cluster 3"=w295, "Target Distance"=13.0) -> ("Cluster 2"=w296:T2)  [unwired: 9 in]
      n131 = call "New PID Move Talon (1).vi"("Cluster 3"=w296, "Target Distance"=7.0 ("Target Angle")) -> ("Cluster 2"=w297:T2)  [unwired: 9 in]
      n132 = call "New PID Move Talon (1).vi"("Cluster 3"=w297, "Target Angle"=90.0 ("Target Distance")) -> ("Cluster 2"=w298:T2)  [unwired: 9 in]
      n133 = call "New PID Move Talon (1).vi"("Cluster 3"=w298, "Target Distance"=1.0) -> ()  [unwired: 9 in, 1 out]
    }
    frame "Middle Right Front Auto" {
      n134 = call "New PID Move Talon (1).vi"("Target Distance"=9.0) -> ()  [unwired: 10 in, 1 out]
    }
    frame "Middle Right Side Auto" {
      n135 = call "New PID Move Talon (1).vi"("Target Distance"=6.0) -> ("Cluster 2"=w307:T2)  [unwired: 10 in]
      n136 = call "New PID Move Talon (1).vi"("Cluster 3"=w307, "Target Angle"=90.0) -> ("Cluster 2"=w308:T2)  [unwired: 9 in]
      n137 = call "New PID Move Talon (1).vi"("Cluster 3"=w308, "Target Distance"=4.0) -> ("Cluster 2"=w309:T2)  [unwired: 9 in]
      n138 = call "New PID Move Talon (1).vi"("Cluster 3"=w309, "Target Angle"=-90.0) -> ("Cluster 2"=w310:T2)  [unwired: 9 in]
      n139 = call "New PID Move Talon (1).vi"("Cluster 3"=w310, "Target Distance"=7.0) -> ("Cluster 2"=w311:T2)  [unwired: 9 in]
      n140 = call "New PID Move Talon (1).vi"("Cluster 3"=w311, "Target Angle"=-90.0) -> ("Cluster 2"=w312:T2)  [unwired: 9 in]
      n141 = call "New PID Move Talon (1).vi"("Cluster 3"=w312, "Target Distance"=1.0) -> ()  [unwired: 9 in, 1 out]
    }
    frame "Middle Left Front Auto" {
      n142 = call "New PID Move Talon (1).vi"("Target Distance"=4.0) -> ("Cluster 2"=w318:T2)  [unwired: 10 in]
      n143 = call "New PID Move Talon (1).vi"("Cluster 3"=w318, "Target Angle"=-90.0) -> ("Cluster 2"=w319:T2)  [unwired: 9 in]
      n144 = call "New PID Move Talon (1).vi"("Cluster 3"=w319, "Target Distance"=9.0) -> ("Cluster 2"=w320:T2)  [unwired: 9 in]
      n145 = call "New PID Move Talon (1).vi"("Cluster 3"=w320, "Target Angle"=90.0) -> ("Cluster 2"=w321:T2)  [unwired: 9 in]
      n146 = call "New PID Move Talon (1).vi"("Cluster 3"=w321, "Target Distance"=5.0) -> ()  [unwired: 9 in, 1 out]
    }
  }
  n147 = disable-structure shown="Disabled" {
    frame Disabled {
      n148 = call "New PID Move Talon (1).vi"("Target Angle"=45.0) -> ("Cluster 2"=w332:T2)  [unwired: 10 in]
      n149 = call "New PID Move Talon (1).vi"("Target Angle"=-45.0) -> ("Cluster 2"=w325:T2)  [unwired: 10 in]
      n150 = Wait (ms)(milliseconds to wait=u32 1000) -> ()  [unwired: 1 out]
      n151 = Wait (ms)(milliseconds to wait=u32 1000) -> ()  [unwired: 1 out]
      n152 = call "New PID Move Talon (1).vi"("Cluster 3"=w325, "Target Distance"=7.0) -> ("Cluster 2"=w324:T2)  [unwired: 9 in]
      n153 = call "New PID Move Talon (1).vi"("Cluster 3"=w332, "Target Distance"=7.0) -> ("Cluster 2"=w331:T2)  [unwired: 9 in]
      n154 = call "New PID Move Talon (1).vi"("Cluster 3"=w331, "Target Angle"=-45.0) -> ("Cluster 2"=w330:T2)  [unwired: 9 in]
      n155 = call "New PID Move Talon (1).vi"("Cluster 3"=w324, "Target Angle"=45.0) -> ("Cluster 2"=w323:T2)  [unwired: 9 in]
      n156 = call "New PID Move Talon (1).vi"("Cluster 3"=w330, "Target Distance"=2.0) -> ()  [unwired: 9 in, 1 out]
      n157 = call "New PID Move Talon (1).vi"("Cluster 3"=w323, "Target Distance"=2.0) -> ()  [unwired: 9 in, 1 out]
    }
    frame Enabled {
    }
  }
  n158 = disable-structure shown="Disabled" {
    frame Disabled {
      # "Old auto programs"
      n159 = call "Auto Move Straight.vi"() -> ()  [unwired: 10 in, 2 out]
      n160 = call "Auto Turn Precise.vi"() -> ()  [unwired: 10 in, 2 out]
    }
    frame Enabled {
    }
  }
  n161 = disable-structure shown="Disabled" {
    frame Disabled {
      n162 = call "New PID Move Talon (1).vi"() -> ()  [unwired: 11 in, 1 out]
    }
    frame Enabled {
    }
  }
  n163 = disable-structure shown="Disabled" {
    frame Disabled {
      n164 = call "Unguided Move (1).vi"() -> ()  [unwired: 11 in, 1 out]
    }
    frame Enabled {
    }
  }
  n165 = disable-structure shown="Disabled" {
    frame Disabled {
      w348 = "Right Intake" ("refnum name")
      w347 = "Left Intake" ("refnum name")
      n166 = call "Unguided Move (1).vi"("Power 2"=0.6, "Power"=0.6, "milliseconds to wait"=u32 2500, "refnum name 2"="Talon1", "refnum name"="Talon4") -> ("error out"=w345:errorcluster)  [unwired: 6 in]
      n167 = call "Unguided Move (1).vi"("Power 2"=-0.75 ("Power"), "Power"=-0.75, "error in (no error)"=w345, "milliseconds to wait"=u32 500, "refnum name 2"=w348, "refnum name"=w347) -> ("error out"=w352:errorcluster)  [unwired: 5 in]
      n168 = call "Unguided Move (1).vi"("Power 2"=-0.75, "Power"=0.75, "error in (no error)"=w352, "milliseconds to wait"=u32 1500, "refnum name 2"=w348, "refnum name"=w347) -> ()  [unwired: 5 in, 1 out]
    }
    frame Enabled {
    }
  }
  n169 = disable-structure shown="Disabled" {
    frame Disabled {
      n170 = for {
        tunnel: [w365] -> _ mode=indexing
        tunnel: [w358] -> _ mode=indexing
        tunnel: _ -> [w359] mode=indexing
        shift-right: [w363] -> _
        shift-left: _ -> [w364]
        shift-right: [w361] -> _
        shift-left: _ -> [w362]
        tunnel: T6 {"Left Encoder"="Talon1", "Right Encoder"="Talon4", "Gyro Refnum"="Gyro", "Device Number"=enum."Dev0", "Right Refnum"="Talon5", "Left Refnum"="Talon2", "Left Intake"="Talon7", "Right Intake"="Talon9"} ("Cluster 3") -> [w354]
        n171 = for {
          N: 100 -> [_]
          tunnel: w359 -> [w431]
          tunnel: [w428] -> w360
          i -> [w428]
          stop <- w427 stop-if-true
          n172 = String Subset(string=w431, offset (0)=w428, length (rest)=1 ("length (rest)")) -> (substring=w429:string)
          n173 = Lexical Class(1:w429) -> (0:w433:i16)
          n174 = Equal?(x=w433, y=i16 3) -> (x = y?=w427:bool)
        }
        n175 = Search/Split String(string=w359, offset (0)=w360) -> (substring before match=w358:string, match + rest of string=w357:string)  [unwired: 1 in, 1 out]
        n176 = Fract/Exp String To Number(string=w357) -> (number=w365:dbl)  [unwired: 3 in, 1 out]
        n177 = case shown="\"R\"" w358 {
          tunnel: w365 -> [w368 w386 w403 w409 w416 w422]
          tunnel: w364 -> [w382 w400 w408 w415 w420 w426]
          tunnel: [w381 w399 w408 w415 w420 w426] -> w363
          tunnel: w362 -> [w375 w393 w406 w413 w419 w425]
          tunnel: [w375 w393 w407 w414 w419 w425] -> w361
          tunnel: i16 10000 ("Timeout") -> [w367 w385 w404 w410 _ _]
          tunnel: w354 -> [w366 w384 w402 _ _ w421]
          frame "F" {
            n178 = expression code="(x/180.0)*pi" "degrees to radians"(w375) -> (w378:dbl)
            n179 = Sine(x=w378) -> (sin(x)=w376:dbl)
            n180 = Cosine(x=w378) -> (cos(x)=w377:dbl)
            n181 = Multiply(x=w368, y=w376) -> (x*y=w380:dbl)
            n182 = Multiply(x=w368, y=w377) -> (x*y=w379:dbl)
            n183 = Multiply(x=1250.0, y=w368) -> (x*y=w371:dbl)
            n184 = Bundle(w380, w379) -> (w372:cluster{dbl, dbl})  [unwired: 1 in]
            n185 = call "New PID Move Talon (1).vi"("Cluster 3"=w366, "Timeout"=w367, "Target Distance"=w371, "Target Angle"=0.0) -> ()  [unwired: 7 in, 1 out]
            n186 = call <vilib>:"Draw Line.vi"("picture"=w382, "end point"=w372, "absolute coordinates?(T)"=FALSE, "color(black)"=u32 6618880, "pen"=T13 {"Width"=2, "Style"=enum."Solid"}) -> ("new picture"=w381:picture)  [unwired: 4 in]
          }
          frame "B" {
            n187 = expression code="(x/180.0)*pi" "degrees to radians"(w393) -> (w396:dbl)
            n188 = Sine(x=w396) -> (sin(x)=w394:dbl)
            n189 = Cosine(x=w396) -> (cos(x)=w395:dbl)
            n190 = Multiply(x=w386, y=w394) -> (x*y=w398:dbl)
            n191 = Multiply(x=w386, y=w395) -> (x*y=w397:dbl)
            n192 = Multiply(x=1250.0, y=w386) -> (x*y=w389:dbl)
            n193 = Bundle(w398, w397) -> (w390:cluster{dbl, dbl})  [unwired: 1 in]
            n194 = call "New PID Move Talon (1).vi"("Cluster 3"=w384, "Timeout"=w385, "Target Distance"=w389, "Target Angle"=0.0) -> ()  [unwired: 7 in, 1 out]
            n195 = call <vilib>:"Draw Line.vi"("picture"=w400, "end point"=w390, "absolute coordinates?(T)"=FALSE, "color(black)"=u32 6618880, "pen"=T13 {"Width"=2, "Style"=enum."Solid"}) -> ("new picture"=w399:picture)  [unwired: 4 in]
          }
          frame "R" {
            n196 = Subtract(x=w406, y=w403) -> (x-y=w407:dbl)
            n197 = call "New PID Move Talon (1).vi"("Cluster 3"=w402, "Timeout"=w404, "Target Distance"=0.0, "Target Angle"=w403) -> ()  [unwired: 7 in, 1 out]
          }
          frame "L" {
            n198 = Negate(x=w409) -> (-x=w412:dbl)
            n199 = call "New PID Move Talon (1).vi"("Timeout"=w410, "Target Distance"=0.0, "Target Angle"=w412) -> ()  [unwired: 8 in, 1 out]
            n200 = Add(x=w413, y=w409) -> (x+y=w414:dbl)
          }
          frame "D", Default {
            n201 = Multiply(x=1000.0, y=w416) -> (x*y=w418:dbl)
            n202 = Wait (ms)(milliseconds to wait=w418) -> ()  [unwired: 1 out]
          }
          frame "C" {
            (unwired) -0.75 ("Power 2")
            (unwired) 0.75 ("Power")
            n203 = Unbundle By Name(w421) -> ("Left Intake"=w424:string, "Right Intake"=w423:string)
            n204 = call "Unguided Move (1).vi"("milliseconds to wait"=w422, "refnum name 2"=w423, "refnum name"=w424) -> ()  [unwired: 8 in, 1 out]
          }
        }
      }
    }
    frame Enabled {
    }
  }
